vi "Cmd Set Command Properties (R).vi"(4 "error in (no error)":errorcluster, 5 "command properties":T1, 7 "command reference":T2) -> (0 "error out":errorcluster, 3 "command reference out":T2)   [LabVIEW 2017, in "NI_Database_API.lvlib"]
doc: "Sets properties on the object as determined by the inputs. This VI works for connections, commands, and parameters. For parameters, a parameter index must be wired to the input below the <B>reference</B>."
uses:
  <vilib>/addons/database/NI_Database_API.lvlib
  <vilib>/addons/database/Command.llb/Cmd ObjectReference.ctl
  <vilib>/addons/database/Command.llb/Cmd Properties.ctl
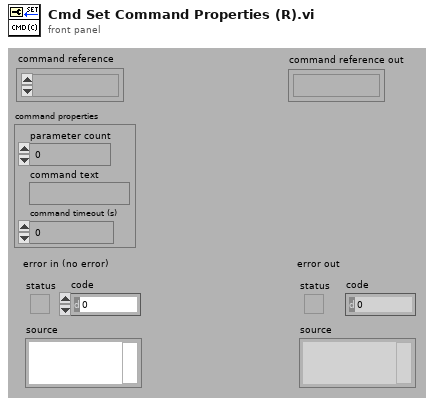
[diagram p1: front panel]
types:
  T1 = typedef "NI_Database_API.lvlib/Cmd Properties.ctl" = cluster{"parameter count":i32, "command text":string, "command timeout (s)":i32}
  T2 = typedef "NI_Database_API.lvlib/Cmd ObjectReference.ctl" = refnum<k1>
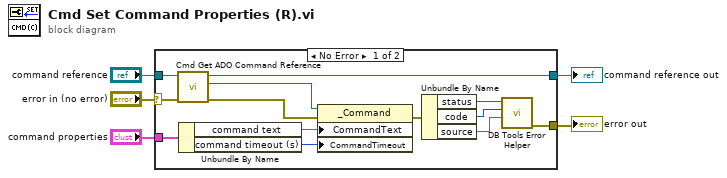
[diagram p0: block diagram]
diagram:
  n1 = case shown="No Error" "error in (no error)" {
    selector: "error in (no error)" -> [w6 w20]
    tunnel: "command reference" -> [w16 w19]
    tunnel: [w15 w19] -> w4
    tunnel: "command properties" -> [w14 _]
    tunnel: [w7 w20] -> w2
    frame No Error {
      n2 = call <vilib>:"Cmd Get ADO Command Reference.vi"("error in (no error)"=w6, "command reference"=w16) -> ("error out"=w17:errorcluster, "ADODB._Command"=w18:refnum<k7>, "command reference out"=w15:T2)  [unwired: 3 out]
      n3 = Unbundle By Name(w14) -> ("command text"=w13:string, "command timeout (s)"=w12:i32)
      n4 = property class="_Command"(reference=w18, error in=w17, "CommandText"=w13, "CommandTimeout"=w12) -> (error out=w8:errorcluster)  [unwired: 1 out]
      n5 = Unbundle By Name(w8) -> ("status"=w10:bool, "code"=w9:i32, "source"=w11:string)
      n6 = call <vilib>:"DB Tools Error Helper.vi"("source"=w11, "code"=w9, "status"=w10) -> ("error out"=w7:errorcluster)  [unwired: 1 in, 7 out]
    }
    frame Error {
    }
  }
  "command reference out" <- w4
  "error out" <- w2
